vi "oa_Calculate Decimation Factor and New Fs.vi"(8 "span":dbl=2000.0, 11 "dt":dbl) -> (1 "new dt":dbl, 2 "decimation factor":i32)   [LabVIEW 2017, in "SoundVib_FaultAnalysis.lvlib"]
uses:
  <vilib>/addons/Sound and Vibration/Order Analysis/Fault Analysis/SoundVib_FaultAnalysis.lvlib
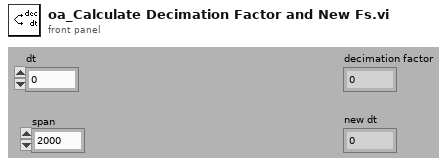
[diagram p1: front panel]
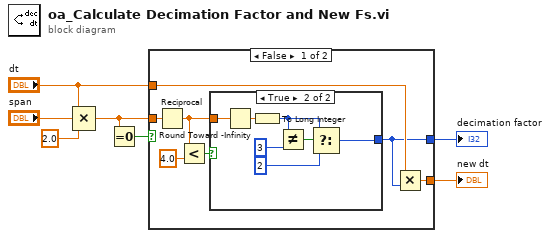
[diagram p0: block diagram]
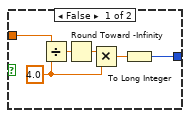
[diagram p2: hidden frame]
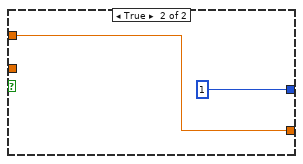
[diagram p3: hidden frame]
diagram:
  n1 = Compound Arithmetic op=MULTIPLY("dt", "span", 2.0 ("value")) -> (w4:dbl)
  n2 = Equal To 0?(x=w4) -> (x = 0?=w5:bool)
  n3 = case shown="False" w5 {
    tunnel: w4 -> [w11 _]
    tunnel: [w8 1] -> w7
    tunnel: [w10 w28] -> w6
    tunnel: "dt" -> [w9 w28]
    frame False {
      n4 = Reciprocal(x=w11) -> (1/x=w12:dbl)
      n5 = Less?(x=w12, y=4.0) -> (x < y?=w13:bool)
      n6 = case shown="True" w13 {
        tunnel: w12 -> [w17 w27]
        tunnel: [w15 w21] -> w8
        frame False {
          w18 = 4.0 ("y")
          n7 = Divide(x=w17, y=w18) -> (x/y=w20:dbl)
          n8 = Round Toward -Infinity(1:w20) -> (0:w19:dbl)
          n9 = Multiply(x=w19, y=w18) -> (x*y=w16:dbl)
          n10 = To Long Integer(number=w16) -> (32bit integer=w15:i32)
        }
        frame True {
          n11 = Round Toward -Infinity(1:w27) -> (0:w26:dbl)
          n12 = To Long Integer(number=w26) -> (32bit integer=w23:i32)
          n13 = Not Equal?(x=w23, y=3) -> (x != y?=w24:bool)
          n14 = Select(t=w23, s=w24, f=2) -> (s? t:f=w21:i32)
        }
      }
      n15 = Multiply(x=w9, y=w8) -> (x*y=w10:dbl)
    }
    frame True {
    }
  }
  "decimation factor" <- w7
  "new dt" <- w6
